vi "Run_1_of_6_Tests.vi"() -> ()   [LabVIEW 2019]
uses:
  <vilib>/Rock Robotics/WPI/ThirdParty/JAS_Junk/TrajLib/Trajectory_Library.lvlib
panel:
  out "Coordinate System":bool
  out "String":string
  out "DC Motor Simulation":bool
  out "Diff Drive Kine Constraint":bool
  out "Diff Drive Voltage Constraint":bool
  out "Bang Bang Input/Output":bool
  out "Bang Bang Tolerance":bool
  out "Debounce":bool
  out "All Tests Finished":bool
  out "Diff Drive Pose Est":bool
  out "Centrip Accel Constraint":bool
  out "Controller Utility":bool
  out "Chassis Speeds":bool
  out "Cubic Spline":bool
  out "Diff Drive Kinematics":bool
  out "Angle Stats":bool
  # "FORMAL TRAJECTORY / CONTROL LIBRARY TEST PROCEDURE"
  # "FUNCTION NOT\nIMPLEMENTED"
  # "Cntrl Affine Plant Inversion"
  # "Diff Drive Odom"
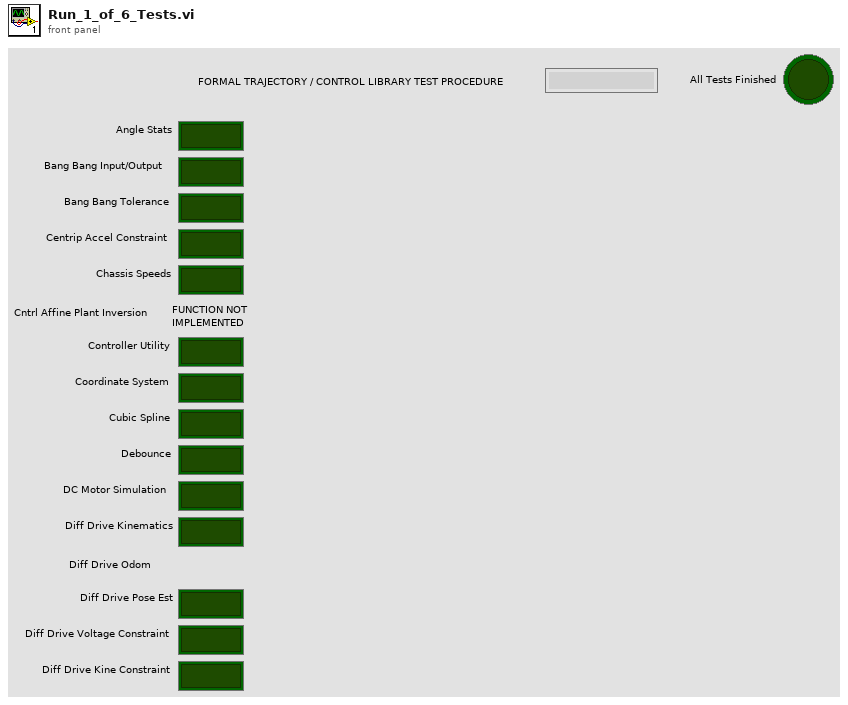
[diagram p1: front panel]
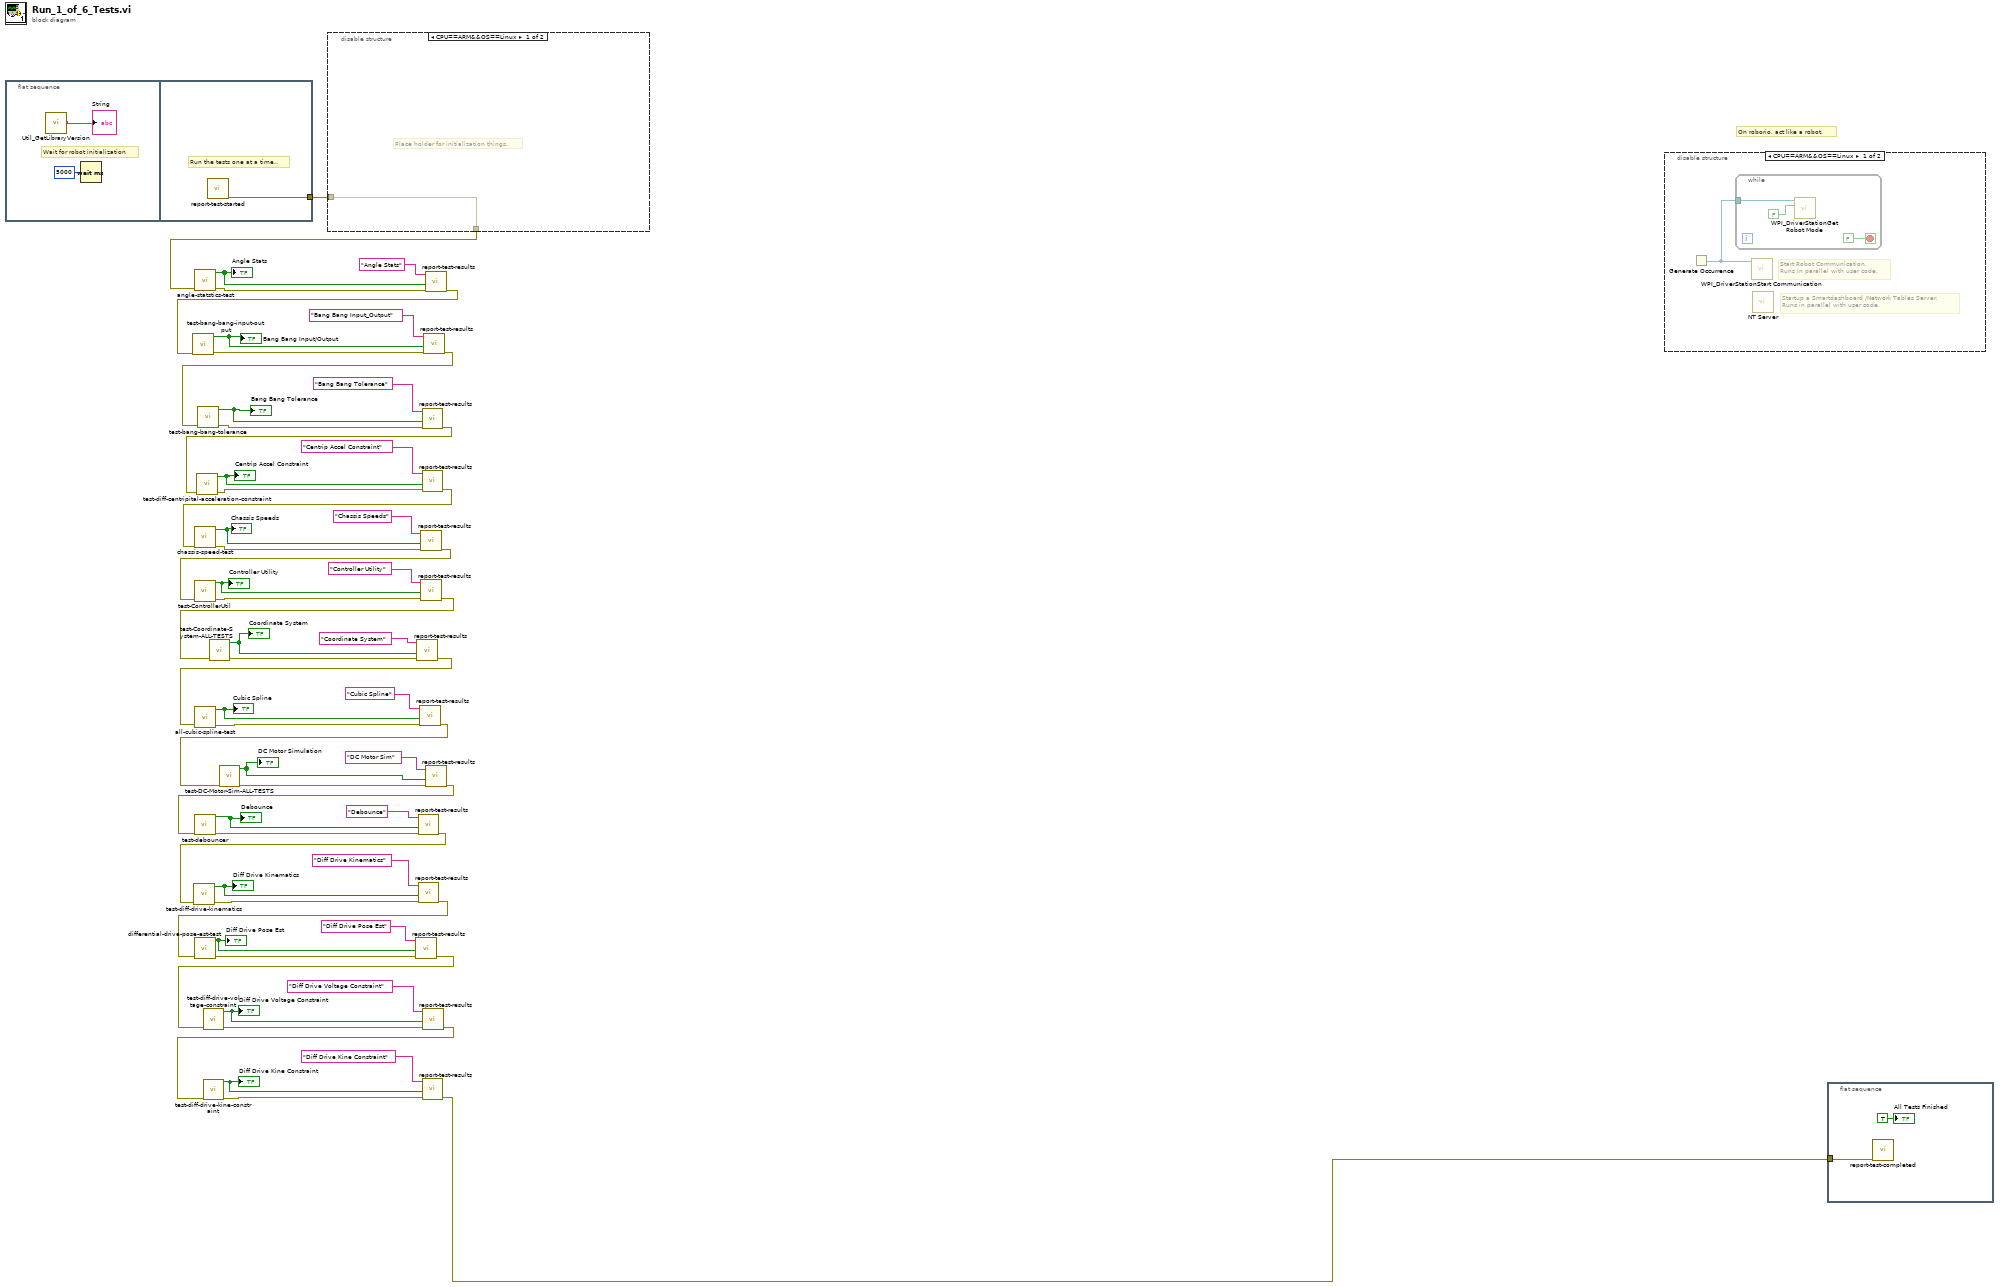
[diagram p0: block diagram]
diagram:
  # "On roborio, act like a robot."
  n1 = flat-sequence {
    tunnel: [w61] -> w21
    frame #0 {
      # "Wait for robot initialization"
      n2 = call <vilib>:"Util_GetLibraryVersion.vi"() -> ("TrajLibVersion"=→"String":string)  [unwired: 11 in]
      n3 = Wait (ms)(milliseconds to wait=u32 5000) -> ()  [unwired: 1 out]
    }
    frame #1 {
      # "Run the tests one at a time.."
      n4 = call "report-test-started.vi"() -> ("error out"=w61:errorcluster)  [unwired: 11 in]
    }
  }
  n5 = disable-structure shown="CPU==ARM&&OS==Linux" {
    disable-tunnel: w21 -> [w62 w63]
    disable-tunnel: [w62 w63] -> w20
    frame condition #0 {
      # "Place holder for initialization things."
    }
    frame condition #1 (active) {
    }
  }
  n6 = call "angle-statstics-test.vi"("error in (no error)"=w20) -> ("error out"=w38:errorcluster, "All Passed"=w58:bool)  [unwired: 9 in]
  "Angle Stats" <- w58
  n7 = call "report-test-results.vi"("error in (no error)"=w38, "TestPassed"=w58, "Test Name"="Angle Stats") -> ("error out"=w37:errorcluster)  [unwired: 8 in]
  n8 = call "test-bang-bang-input-output.vi"("error in (no error)"=w37) -> ("error out"=w36:errorcluster, "All Tests Passed"=w55:bool)  [unwired: 9 in]
  "Bang Bang Input/Output" <- w55
  n9 = call "report-test-results.vi"("error in (no error)"=w36, "TestPassed"=w55, "Test Name"="Bang Bang Input_Output") -> ("error out"=w35:errorcluster)  [unwired: 8 in]
  n10 = call "test-bang-bang-tolerance.vi"("error in (no error)"=w35) -> ("error out"=w34:errorcluster, "All Tests Passed"=w53:bool)  [unwired: 9 in]
  "Bang Bang Tolerance" <- w53
  n11 = call "report-test-results.vi"("error in (no error)"=w34, "TestPassed"=w53, "Test Name"="Bang Bang Tolerance") -> ("error out"=w33:errorcluster)  [unwired: 8 in]
  n12 = call "test-diff-centripital-acceleration-constraint.vi"("error in (no error)"=w33) -> ("error out 2"=w32:errorcluster, "Test Passed"=w51:bool)  [unwired: 9 in]
  "Centrip Accel Constraint" <- w51
  n13 = call "report-test-results.vi"("error in (no error)"=w32, "TestPassed"=w51, "Test Name"="Centrip Accel Constraint") -> ("error out"=w31:errorcluster)  [unwired: 8 in]
  n14 = call "chassis-speed-test.vi"("error in (no error)"=w31) -> ("error out"=w30:errorcluster, "Test Passed"=w49:bool)  [unwired: 9 in]
  "Chassis Speeds" <- w49
  n15 = call "report-test-results.vi"("error in (no error)"=w30, "TestPassed"=w49, "Test Name"="Chassis Speeds") -> ("error out"=w29:errorcluster)  [unwired: 8 in]
  n16 = call "test-ControllerUtil.vi"("error in (no error)"=w29) -> ("error out"=w28:errorcluster, "All Tests Passed"=w47:bool)  [unwired: 9 in]
  "Controller Utility" <- w47
  n17 = call "report-test-results.vi"("error in (no error)"=w28, "TestPassed"=w47, "Test Name"="Controller Utility") -> ("error out"=w2:errorcluster)  [unwired: 8 in]
  n18 = call "test-Coordinate-System-ALL-TESTS.vi"("error in (no error)"=w2) -> ("error out"=w4:errorcluster, "All Passed"=w3:bool)  [unwired: 9 in]
  "Coordinate System" <- w3
  n19 = call "report-test-results.vi"("error in (no error)"=w4, "TestPassed"=w3, "Test Name"="Coordinate System") -> ("error out"=w1:errorcluster)  [unwired: 8 in]
  n20 = call "all-cubic-spline-test.vi"("error in (no error)"=w1) -> ("error out"=w27:errorcluster, "ALL TESTS PASSED"=w43:bool)  [unwired: 9 in]
  "Cubic Spline" <- w43
  n21 = call "report-test-results.vi"("error in (no error)"=w27, "TestPassed"=w43, "Test Name"="Cubic Spline") -> ("error out"=w7:errorcluster)  [unwired: 8 in]
  n22 = call "test-DC-Motor-Sim-ALL-TESTS.vi"("error in (no error)"=w7) -> ("error out"=w9:errorcluster, "All Passed"=w8:bool)  [unwired: 9 in]
  "DC Motor Simulation" <- w8
  n23 = call "report-test-results.vi"("error in (no error)"=w9, "TestPassed"=w8, "Test Name"="DC Motor Sim") -> ("error out"=w6:errorcluster)  [unwired: 8 in]
  n24 = call "test-debouncer.vi"("error in (no error)"=w6) -> ("error out"=w26:errorcluster, "ALL TESTS PASSED"=w42:bool)  [unwired: 9 in]
  "Debounce" <- w42
  n25 = call "report-test-results.vi"("error in (no error)"=w26, "TestPassed"=w42, "Test Name"="Debounce") -> ("error out"=w22:errorcluster)  [unwired: 8 in]
  n26 = call "test-diff-drive-kinematics.vi"("error in (no error)"=w22) -> ("error out"=w25:errorcluster, "All Passed"=w41:bool)  [unwired: 9 in]
  "Diff Drive Kinematics" <- w41
  n27 = call "report-test-results.vi"("error in (no error)"=w25, "TestPassed"=w41, "Test Name"="Diff Drive Kinematics") -> ("error out"=w23:errorcluster)  [unwired: 8 in]
  n28 = call "differential-drive-pose-est-test.vi"("error in (no error)"=w23) -> ("error out"=w24:errorcluster, "Test Passed"=w39:bool)  [unwired: 9 in]
  "Diff Drive Pose Est" <- w39
  n29 = call "report-test-results.vi"("error in (no error)"=w24, "TestPassed"=w39, "Test Name"="Diff Drive Pose Est") -> ("error out"=w16:errorcluster)  [unwired: 8 in]
  n30 = call "test-diff-drive-voltage-constraint.vi"("error in (no error)"=w16) -> ("error out 4"=w17:errorcluster, "Test Passed"=w18:bool)  [unwired: 9 in]
  "Diff Drive Voltage Constraint" <- w18
  n31 = call "report-test-results.vi"("error in (no error)"=w17, "TestPassed"=w18, "Test Name"="Diff Drive Voltage Constraint") -> ("error out"=w12:errorcluster)  [unwired: 8 in]
  n32 = call "test-diff-drive-kine-constraint.vi"("error in (no error)"=w12) -> ("error out 2"=w13:errorcluster, "Test Passed"=w14:bool)  [unwired: 9 in]
  "Diff Drive Kine Constraint" <- w14
  n33 = call "report-test-results.vi"("error in (no error)"=w13, "TestPassed"=w14, "Test Name"="Diff Drive Kine Constraint") -> ("error out"=w11:errorcluster)  [unwired: 8 in]
  n34 = disable-structure shown="CPU==ARM&&OS==Linux" {
    frame condition #0 {
      # "Startup a Smartdashboard /Network Tables Server.\nRuns in parallel with user code."
      # "Start Robot Communication.\nRuns in parallel with user code."
      n35 = Generate Occurrence() -> (w64:refnum<k4>)
      n36 = while {
        tunnel: w64 -> [w67]
        stop <- FALSE stop-if-true
        n37 = call <vilib>:"WPI_DriverStationGet Robot Mode.vi"("Finish"=FALSE, "DS Occurrence"=w67) -> ()  [unwired: 10 out]
      }
      n38 = call <vilib>:"WPI_DriverStationStart Communication.vi"("occurrence"=w64) -> ()  [unwired: 2 in, 9 out]
      n39 = call <vilib>:"NT Server.vi"() -> ()  [unwired: 12 in]
    }
    frame condition #1 (active) {
    }
  }
  n40 = flat-sequence {
    tunnel: w11 -> [w68]
    frame #0 {
      n41 = call "report-test-completed.vi"("error in (no error)"=w68) -> ()  [unwired: 10 in, 1 out]
      "All Tests Finished" <- TRUE ("All Tests Finished")
    }
  }
